vi "Image_Processing_Queue.vi"(5 "Data":T4={"L16 Linear Actuator"="", "XE 1000 Pump"="", "Camera1"="", "Camera2"="", "Camera1_IMG"=refnum, "Camera2_IMG"=refnum, "Img_Capt"=FALSE, "Actuator"=FALSE, "Pump"=FALSE, "Cam 1"=FALSE, "Cam 2"=FALSE, "Empty_Refill"=FALSE, "Crop"=FALSE, "Light intensity"=100, "Exposure Time"=1000.0, "Sample Name"="Test Sample", "Operator"="MRJ", "Calibration 1"=path "C:/Users/au540322/Desktop/IHS_Project/images/Debris/Debris_0/Debris_0_2019_06_01-23-32-49-686.PNG", "Calibration 2"=path "C:/Users/au540322/Desktop/IHS_Project/images/Debris/Debris_0/Debris_0_2019_06_01-23-32-49-686.PNG", "Framerate"=1, "Timeout Sample"=0, "Collection date"="MRJ", "Sample size threshold"=1, "Empty start"=1, "Command"="MRJ", "Calibration Image 1"=refnum, "Calibration Image 2"=refnum, "Original Image 1"=refnum, "Original Image 2"=refnum, "Processing Image 1"=refnum, "Processing Image 2"=refnum, "Object Image 1"=refnum, "Object Image 2"=refnum, "Cam 1 - save queue"=refnum, "Cam 2 - save queue"=refnum, "Station"="", "Species Name"="", "Other Notes"="", "Aperture"=enum."Item 0", "Image Process Queue Size"=500, "Image Save Queue Size"=500, "Overload threshold"=500, "Max Framerate"=100, "Blue Plane Image"=refnum, "Subtract Image"=refnum, "Binary Image 1"=refnum, "ROI mask allocation"=refnum, "Rectangle 1"={"Left"=0, "Top"=0, "Right"=0, "Bottom"=0, "Rotation"=0.0}, "Rectangle 2"={"Left"=0, "Top"=0, "Right"=0, "Bottom"=0, "Rotation"=0.0}, "Binary Image 2"=refnum, "Detection Region %"=0.0, "Cam 1 queue"=refnum, "Cam 2 queue"=refnum, "Detect image 1"=refnum, "Detect image 2"=refnum, "Detect 1"=path "C:/Users/au540322/Desktop/IHS_Project/images/Debris/Debris_0/Debris_0_2019_06_01-23-32-49-686.PNG", "Detect 2"=path "C:/Users/au540322/Desktop/IHS_Project/images/Debris/Debris_0/Debris_0_2019_06_01-23-32-49-686.PNG", "Max large object threshold"=0, "Open(T)/Close(F)"=FALSE} {"Rectangle 2"."Rotation" format="%.2f"; "Rectangle 2"."Left" scale=0.0..1024.0; "Rectangle 2"."Right" scale=0.0..1024.0; "Rectangle 1"."Rotation" format="%.2f"; "Rectangle 1"."Left" scale=0.0..1024.0; "Rectangle 1"."Right" scale=0.0..1024.0; "Max Framerate" min=1; "Overload threshold" min=1; "Image Save Queue Size" min=1; "Image Process Queue Size" min=1; "Empty start" min=1; "Sample size threshold" min=1; "Framerate" min=1; "Light intensity" scale=0.0..100.0}) -> (10 "Status":T1, 12 "Process queue":T2, 13 "Last Image?":bool, 14 "Object1":T3, 15 "Object2":T3, 16 "Image 1":T3, 17 "Image 2":T3, 18 "Binary 1":T3, 19 "Binary 2":T3)   [LabVIEW 2019]
doc: "Saves every 6th image in a sub folder in the current directory (specified from Sample Name). When a true is sent to Sample+1 a new subfolder is created with incremental numbering.\nExample of folders: \n../images/Sample_Name/Sample_Name1\n../images/Sample_Name/Sample_Name2"
uses:
  controls/Data.ctl
  <vilib>/userdefined/High Color/IMAQdx.ctl
  <vilib>/vision/Image Controls.llb/IMAQ Image.ctl
  <extravilib>/ChannelInstances/Tag-c(bool,bool)/))Channel.ctl
  Camera_ID.ctl
  <extravilib>/ChannelInstances/Tag-c(bool,bool)/Write With Abort.vi
  <extravilib>/ChannelInstances/Tag-c(bool,bool)/Endpoint.vi
  <extravilib>/ChannelInstances/Tag-c(bool,bool).lvlib
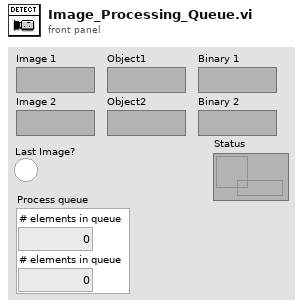
[diagram p1: front panel]
types:
  T1 = typedef "Tag-c(bool,bool).lvlib/))Channel.ctl" = refnum<queue>
  T2 = cluster{"# elements in queue":i32, "# elements in queue":i32}
  T3 = typedef "IMAQ Image.ctl" = refnum<image>
  T4 = typedef "Data.ctl" = cluster{"L16 Linear Actuator":refnum<visa-resource-name>, "XE 1000 Pump":refnum<visa-resource-name>, "Camera1":T5, "Camera2":T5, "Camera1_IMG":T3, "Camera2_IMG":T3, "Img_Capt":bool, "Actuator":bool, "Pump":bool, "Cam 1":bool, "Cam 2":bool, "Empty_Refill":bool, "Crop":bool, "Light intensity":i32, "Exposure Time":dbl, "Sample Name":string, "Operator":string, "Calibration 1":path, "Calibration 2":path, "Framerate":i32, "Timeout Sample":i32, "Collection date":string, "Sample size threshold":i32, "Empty start":u32, "Command":string, "Calibration Image 1":T3, "Calibration Image 2":T3, "Original Image 1":T3, "Original Image 2":T3, "Processing Image 1":T3, "Processing Image 2":T3, "Object Image 1":T3, "Object Image 2":T3, "Cam 1 - save queue":refnum<queue>, "Cam 2 - save queue":refnum<queue>, "Station":string, "Species Name":string, "Other Notes":string, "Aperture":enum32{"Item 0", "Item 1", "Item 2", "Item 3"}, "Image Process Queue Size":i32, "Image Save Queue Size":i32, "Overload threshold":i32, "Max Framerate":i32, "Blue Plane Image":T3, "Subtract Image":T3, "Binary Image 1":T3, "ROI mask allocation":T3, "Rectangle 1":T6, "Rectangle 2":T6, "Binary Image 2":T3, "Detection Region %":dbl, "Cam 1 queue":refnum<queue>, "Cam 2 queue":refnum<queue>, "Detect image 1":T3, "Detect image 2":T3, "Detect 1":path, "Detect 2":path, "Max large object threshold":i32, "Open(T)/Close(F)":bool}
  T5 = typedef "IMAQdx.ctl" = refnum<k21>
  T6 = typedef "IMAQ Rectangle" = cluster{"Left":i32, "Top":i32, "Right":i32, "Bottom":i32, "Rotation":dbl}
  T7 = typedef "Camera_ID.ctl" = enum16{"Camera 1", "Camera 2"}
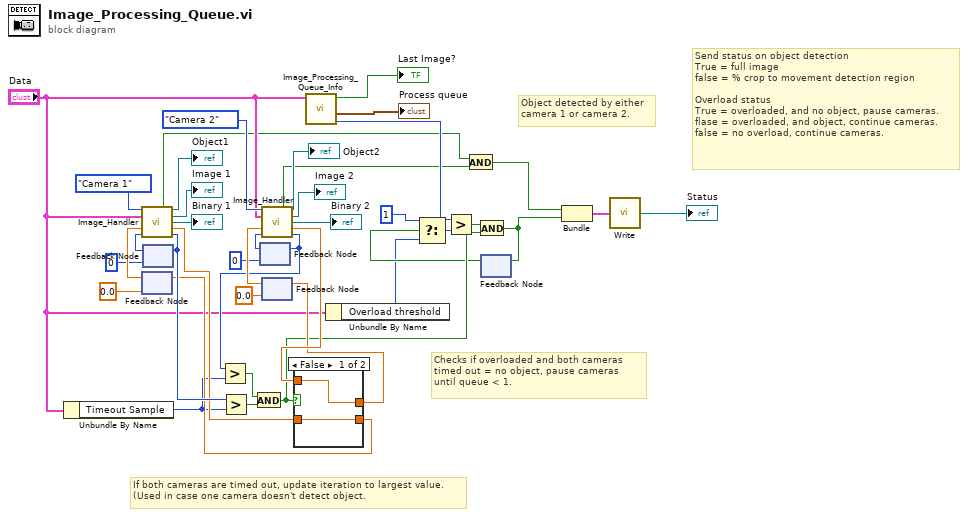
[diagram p0: block diagram]
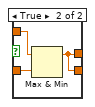
[diagram p2: hidden frame]
diagram:
  # "Send status on object detection\nTrue = full image\nfalse = % crop to movement detection region\n\nOverload status\nTrue = overloaded, and no object, pause cameras.\nflase = overloaded, and object, continue cameras.\nfalse = no overload, continue cameras."
  # "Object detected by either\ncamera 1 or camera 2."
  # "Checks if overloaded and both cameras \ntimed out = no object, pause cameras \nuntil queue < 1."
  # "If both cameras are timed out, update iteration to largest value.\n(Used in case one camera doesn't detect object."
  n1 = Unbundle By Name("Data") -> ("Timeout Sample"=w17:i32)
  n2 = feedback #1(0.0 ("Sample nr")) -> (w32:dbl)
  n3 = feedback #2(0 ("Timeout out")) -> (w30:i32)
  n4 = call "Image_Handler.vi"("Camera"=Camera_ID."Camera 1", "Data"="Data", "Prev. sample"=w32, "Timeout in"=w30) -> ("Object"=w3:bool, "Detected object"=→"Object1":T3, "Image Out"=→"Image 1":T3, "Binary"=→"Binary 1":T3, "Sample nr"=w22:dbl, "Timeout out"=w24:i32)  [unwired: 6 in]
  n5 = feedback-in #2(w24) -> ()
  n6 = Greater?(x=w24, y=w17) -> (0:w21:bool)
  n7 = feedback #3(0 ("Timeout out")) -> (w29:i32)
  n8 = feedback #4(0.0 ("Sample nr")) -> (w31:dbl)
  n9 = call "Image_Handler.vi"("Camera"=Camera_ID."Camera 2", "Data"="Data", "Prev. sample"=w31, "Timeout in"=w29) -> ("Object"=w4:bool, "Detected object"=→"Object2":T3, "Image Out"=→"Image 2":T3, "Binary"=→"Binary 2":T3, "Sample nr"=w23:dbl, "Timeout out"=w18:i32)  [unwired: 6 in]
  n10 = Greater?(x=w18, y=w17) -> (0:w16:bool)
  n11 = And(x=w16, y=w21) -> (x .and. y?=w13:bool)
  n12 = feedback-in #3(w18) -> ()
  n13 = case shown="False" w13 {
    tunnel: w23 -> [w43 w46]
    tunnel: w22 -> [w42 w45]
    tunnel: [w43 w44] -> w20
    tunnel: [w42 w44] -> w19
    frame False {
    }
    frame True {
      n14 = Max & Min(x=w46, y=w45) -> (max(x,y)=w44:dbl)  [unwired: 1 out]
    }
  }
  n15 = feedback-in #1(w19) -> ()
  n16 = feedback-in #4(w20) -> ()
  n17 = call "Image_Processing_Queue_Info.vi"("Data"="Data") -> ("Max Queue Size"=w9:i32, "Queue data"=→"Process queue":T2, "Last Image?"=→"Last Image?":bool)  [unwired: 8 in]
  n18 = Unbundle By Name("Data") -> ("Overload threshold"=w8:i32)
  n19 = And(x=w3, y=w4) -> (x .and. y?=w5:bool)
  n20 = feedback #5() -> (w11:bool)  [unwired: 1 in]
  n21 = Select(t=1 ("y"), s=w11, f=w8) -> (s? t:f=w10:i32)
  n22 = Greater?(x=w9, y=w10) -> (0:w14:bool)
  n23 = And(x=w14, y=w13) -> (x .and. y?=w6:bool)
  n24 = feedback-in #5(w6) -> ()
  n25 = Bundle(w5, w6) -> (w2:cluster{bool, bool})  [unwired: 1 in]
  n26 = call <extravilib>:"Write.vi"("element"=w2) -> ("channel"=→"Status":T1)  [unwired: 1 out]
